vi "update.start_time.request.vi"(8 "error in":errorcluster, 11 "start time":timestamp format="%<%x %.3X>T") -> (0 "error out":errorcluster, 1 "Request":string)   [LabVIEW 2020, in "Run.lvclass"]
uses:
  a758d7e6-d810-4ac6-bb20-f62cb1c30fdd.vi
  <vilib>/LabVIEW Open Source Project/Epoch Date & Time/epoch.UNIX/Epoch.UNIX.lvclass
  C:/Program Files/National Instruments/LabVIEW 2020/vi.lib/LabVIEW Open Source Project/Epoch Date & Time/epoch/Epoch.lvclass
  <vilib>/LabVIEW Open Source Project/Epoch Date & Time/Get Epoch Time.vi
  Run.lvclass
  Run.lvclass/Run.ctl
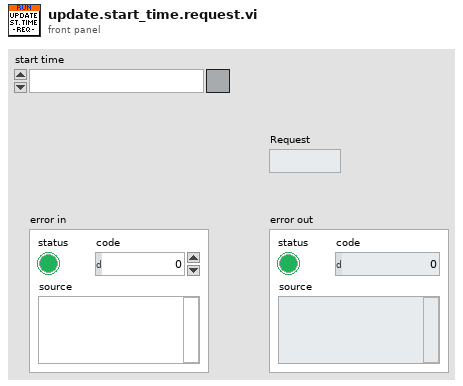
[diagram p1: front panel]
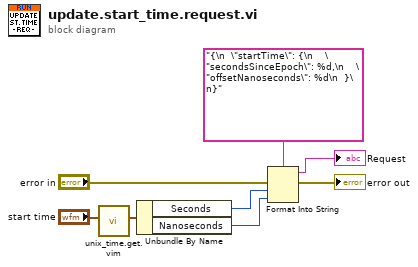
[diagram p0: block diagram]
diagram:
  n1 = call "unix_time.get.vim"("Time Stamp (empty: now) [single or array]"="start time") -> ("UNIX Timestamp"=w4:cluster{"Seconds":i64, "Nanoseconds":i64})  [unwired: 10 in]
  n2 = Unbundle By Name(w4) -> ("Seconds"=w3:i64, "Nanoseconds"=w2:i64)
  n3 = Format Into String(format string="{\n  \"startTime\": {\n    \"secondsSinceEpoch\": %d,\n    \"offsetNanoseconds\": %d\n  }\n}", error in="error in", w3, w2) -> (resulting string=→"Request":string, error out=→"error out":errorcluster)  [unwired: 1 in]
